vi "SampleGetPositionAllSlaves_8742.vi"() -> ()   [LabVIEW 2009]
panel:
  out "Output:":string
  out "DeviceKey List Out":string[](array[string])
  out "error out":errorcluster
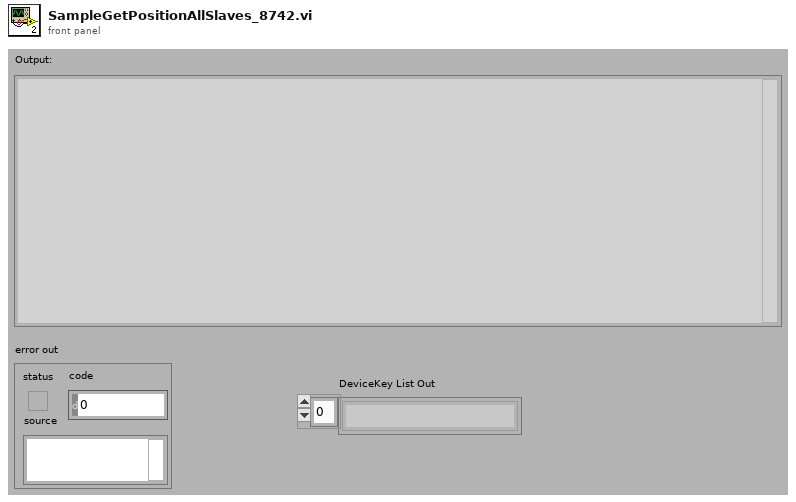
[diagram p1: front panel]
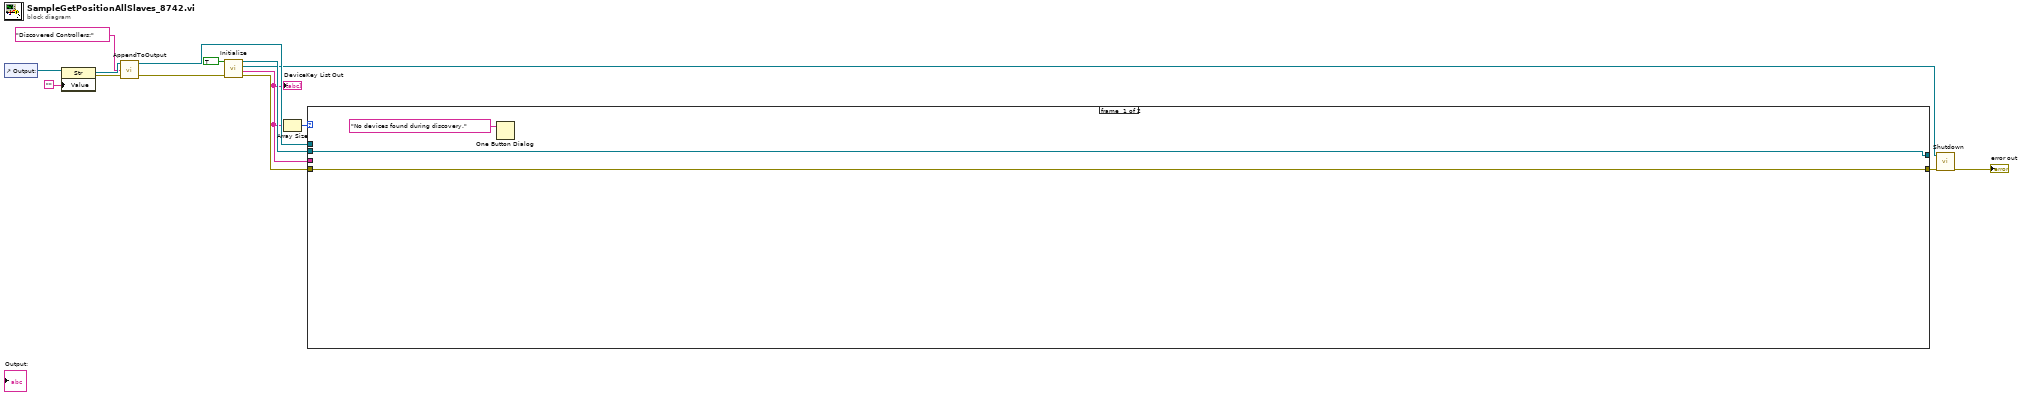
[diagram p0: block diagram]
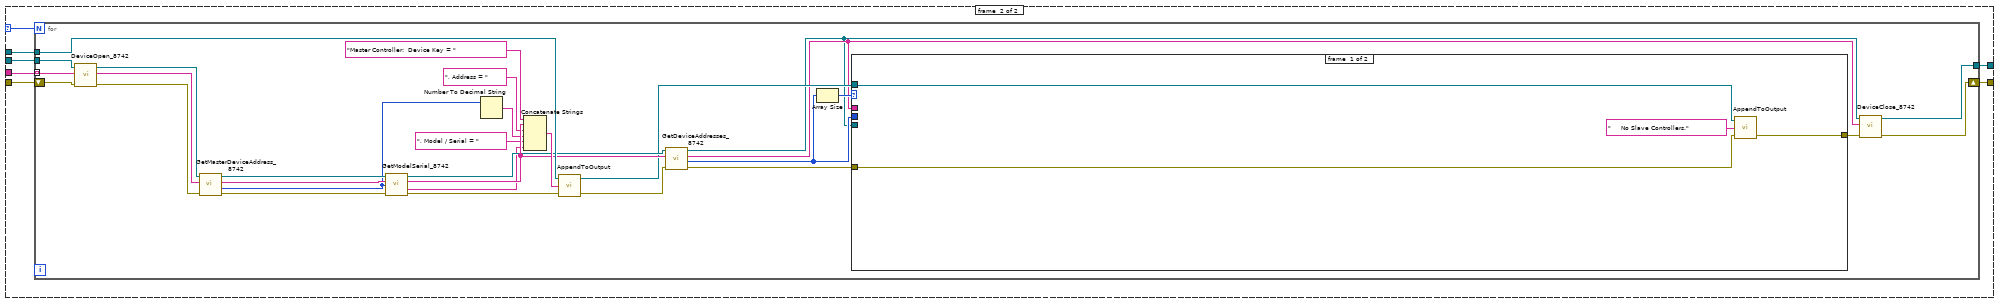
[diagram p2: hidden frame]
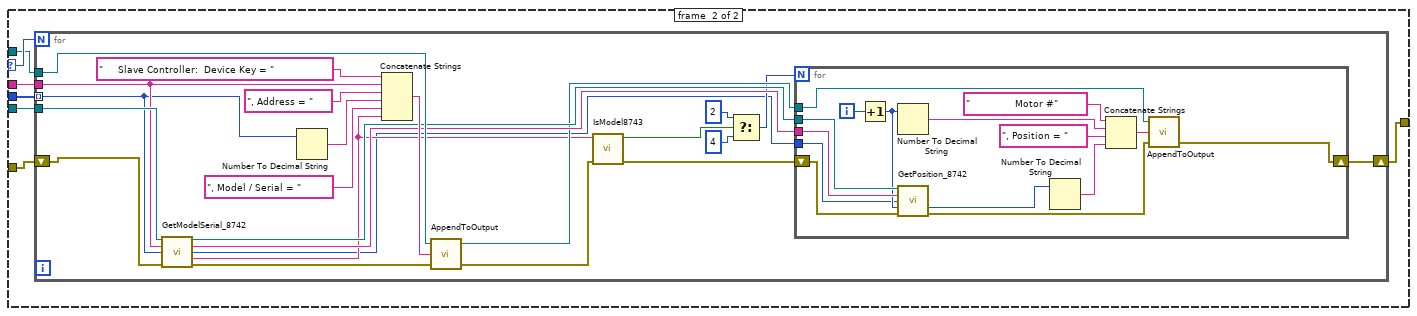
[diagram p3: hidden frame]
diagram:
  n1 = control-ref of="Output:"() -> (w9:refnum<vi>)
  n2 = property class="Str"(reference=w9, "Value"="") -> (reference out=w7:refnum<vi>, error out=w6:errorcluster)  [unwired: 1 in]
  n3 = call "AppendToOutput.vi"("error in"=w6, "Input String"="Discovered Controllers:", "Output Refnum In"=w7) -> ("error out"=w5:errorcluster, "Output Refnum Out"=w3:refnum<vi>)  [unwired: 1 in]
  n4 = call "Initialize.vi"("error in (no error)"=w5, "logging"=TRUE) -> ("error out"=w11:errorcluster, "DeviceKey List"=w2:string[], "DeviceIOLib Out"=w1:refnum<k24>, "CmdLib Out"=w12:refnum<k24>)  [unwired: 2 in]
  "DeviceKey List Out" <- w2
  n5 = Array Size(array=w2) -> (size(s)=w13:i32)
  n6 = case shown="1, Default" w13 {
    selector: w13 -> [_ w25]
    tunnel: w2 -> [_ w24]
    tunnel: w12 -> [w17 w23]
    tunnel: w11 -> [w18 w22]
    tunnel: [w18 w19] -> w10
    tunnel: [w17 w21] -> _
    tunnel: w3 -> [_ w20]
    frame #0 {
      n7 = One Button Dialog(message="No devices found during discovery.") -> ()  [unwired: 1 in, 1 out]
    }
    frame #1 {
      n8 = for {
        N: w25 -> [_]
        tunnel: w24 -> [w53] mode=indexing
        tunnel: w23 -> [w55]
        tunnel: [w54] -> w21
        tunnel: w20 -> [w51]
        shift-right: [w27] -> w19
        shift-left: w22 -> [w52]
        n9 = call "DeviceOpen_8742.vi"("error in (no error)"=w52, "DeviceKey In"=w53, "CmdLib In"=w55) -> ("error out"=w45:errorcluster, "DeviceKey Out"=w46:string, "CmdLib Out"=w47:refnum<k24>)  [unwired: 2 in]
        n10 = call "GetMasterDeviceAddress_8742.vi"("error in (no error)"=w45, "DeviceKey In"=w46, "CmdLib In"=w47) -> ("error out"=w42:errorcluster, "Device Address"=w26:i32, "DeviceKey Out"=w41:string, "CmdLib Out"=w40:refnum<k24>)  [unwired: 1 in]
        n11 = call "GetModelSerial_8742.vi"("CmdLib In"=w40, "DeviceKey In"=w41, "Device Address In"=w26, "error in (no error)"=w42) -> ("CmdLib Out"=w43:refnum<k24>, "DeviceKey Out"=w39:string, "Model / Serial"=w35:string, "error out"=w44:errorcluster)  [unwired: 7 in, 1 out]
        n12 = Number To Decimal String(number=w26) -> (decimal integer string=w37:string)  [unwired: 1 in]
        n13 = Concatenate Strings("Master Controller:  Device Key = " ("string"), w39, ", Address = " ("string"), w37, ", Model / Serial = " ("string"), w35) -> (w50:string)
        n14 = call "AppendToOutput.vi"("error in"=w44, "Input String"=w50, "Output Refnum In"=w51) -> ("error out"=w48:errorcluster, "Output Refnum Out"=w33:refnum<vi>)  [unwired: 1 in]
        n15 = call "GetDeviceAddresses_8742.vi"("error in (no error)"=w48, "DeviceKey In"=w39, "CmdLib In"=w43) -> ("error out"=w32:errorcluster, "Device Addresses"=w30:i32[], "DeviceKey Out"=w29:string, "CmdLib Out"=w28:refnum<k24>)  [unwired: 1 in]
        n16 = Array Size(array=w30) -> (size(s)=w34:i32)
        n17 = case shown="1, Default" w34 {
          selector: w34 -> [_ w66]
          tunnel: w33 -> [w58 w62]
          tunnel: w32 -> [w57 w60]
          tunnel: [w56 w63] -> w31
          tunnel: w30 -> [_ w65]
          tunnel: w29 -> [_ w64]
          tunnel: w28 -> [_ w61]
          frame #0 {
            n18 = call "AppendToOutput.vi"("error in"=w57, "Input String"="     No Slave Controllers.", "Output Refnum In"=w58) -> ("error out"=w56:errorcluster)  [unwired: 1 in, 1 out]
          }
          frame #1 {
            n19 = for {
              N: w66 -> [_]
              tunnel: w65 -> [w81] mode=indexing
              tunnel: w64 -> [w82]
              tunnel: w62 -> [w85]
              tunnel: w61 -> [w83]
              shift-right: [w77] -> w63
              shift-left: w60 -> [w80]
              n20 = call "GetModelSerial_8742.vi"("CmdLib In"=w83, "DeviceKey In"=w82, "Device Address In"=w81, "error in (no error)"=w80) -> ("CmdLib Out"=w78:refnum<k24>, "DeviceKey Out"=w79:string, "Device Address Out"=w67:i32, "Model / Serial"=w70:string, "error out"=w75:errorcluster)  [unwired: 7 in]
              n21 = Number To Decimal String(number=w81) -> (decimal integer string=w87:string)  [unwired: 1 in]
              n22 = Concatenate Strings("     Slave Controller:  Device Key = " ("string"), w82, ", Address = " ("string"), w87, ", Model / Serial = " ("string"), w70) -> (w84:string)
              n23 = call "AppendToOutput.vi"("error in"=w75, "Input String"=w84, "Output Refnum In"=w85) -> ("error out"=w69:errorcluster, "Output Refnum Out"=w76:refnum<vi>)  [unwired: 1 in]
              n24 = call "IsModel8743.vi"("error in"=w69, "Model / Serial"=w70) -> ("error out"=w68:errorcluster, "Boolean"=w74:bool)  [unwired: 8 in]
              n25 = Select(t=2, s=w74, f=4) -> (s? t:f=w71:i32)
              n26 = for {
                N: w71 -> [_]
                tunnel: w79 -> [w104]
                tunnel: w78 -> [w103]
                tunnel: w76 -> [w100]
                shift-right: [w101] -> w77
                shift-left: w68 -> [w102]
                tunnel: w67 -> [w90]
                i -> [w96]
                n27 = Increment(x=w96) -> (x+1=w92:i32)
                n28 = Number To Decimal String(number=w92) -> (decimal integer string=w97:string)  [unwired: 1 in]
                n29 = call "GetPosition_8742.vi"("CmdLib In"=w103, "DeviceKey In"=w104, "Device Address In"=w90, "Motor"=w92, "error in (no error)"=w102) -> ("Position"=w95:i32, "error out"=w91:errorcluster)  [unwired: 6 in, 3 out]
                n30 = Number To Decimal String(number=w95) -> (decimal integer string=w94:string)  [unwired: 1 in]
                n31 = Concatenate Strings("               Motor #" ("Input String"), w97, ", Position = " ("string"), w94) -> (w98:string)
                n32 = call "AppendToOutput.vi"("error in"=w91, "Input String"=w98, "Output Refnum In"=w100) -> ("error out"=w101:errorcluster)  [unwired: 1 in, 1 out]
              }
            }
          }
        }
        n33 = call "DeviceClose_8742.vi"("error in (no error)"=w31, "DeviceKey In"=w29, "CmdLib In"=w28) -> ("error out"=w27:errorcluster, "CmdLib Out"=w54:refnum<k24>)  [unwired: 2 in, 1 out]
      }
    }
  }
  n34 = call "Shutdown.vi"("error in (no error)"=w10, "DeviceIOLib In"=w1) -> ("error out"=→"error out":errorcluster)  [unwired: 5 in]
